vi "Scale Image.vi"(8 "error in (no error)":errorcluster, 11 "EmbedImage in":refnum<class "EmbedImage.lvclass">) -> (0 "error out":errorcluster, 3 "EmbedImage out":refnum<class "EmbedImage.lvclass">)   [LabVIEW 2023, in "EmbedImage.lvlib" / "EmbedImage.lvclass"]
uses:
  Library/EmbedImage.lvclass
  Library/EmbedImage.lvclass/EmbedImage.ctl
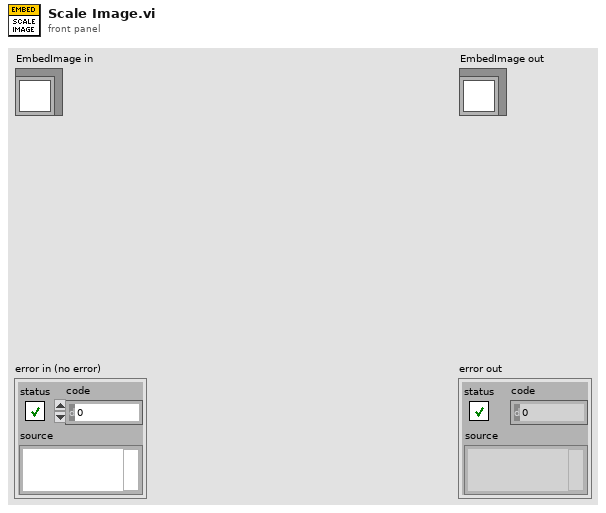
[diagram p1: front panel]
types:
  T1 = typedef "imagedata.ctl" = cluster{"image type":i32, "image depth":i32, "image":u8[], "mask":u8[], "colors":u32[], "Rectangle":cluster{"left":i16, "top":i16, "right":i16, "bottom":i16}}
  T2 = typedef "LVBoundsTypeDef.ctl" = cluster{"Width":u32, "Height":u32}
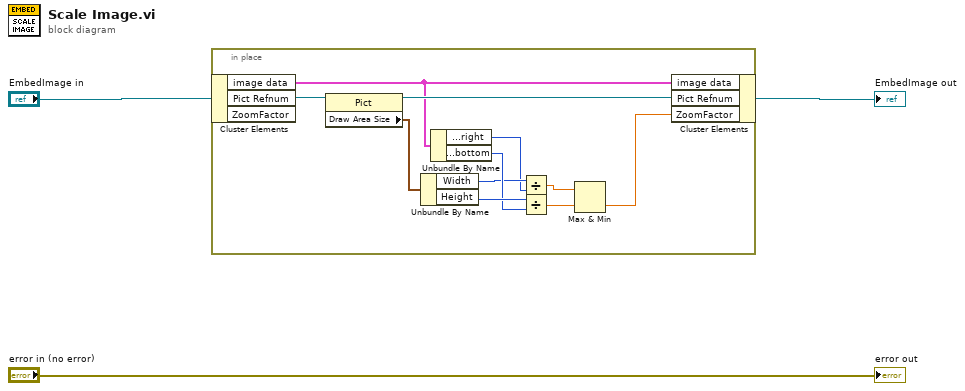
[diagram p0: block diagram]
diagram:
  n1 = in-place {
    n2 = in-place-cluster #1("EmbedImage in") -> ("image data"=w11:T1, "Pict Refnum"=w14:refnum<vi>)  [unwired: 1 out]
    n3 = property class="Pict"(reference=w14) -> (reference out=w13:refnum<vi>, "Draw Area Size"=w12:T2)  [unwired: 1 in, 1 out]
    n4 = Unbundle By Name(w12) -> ("Width"=w8:u32, "Height"=w10:u32)
    n5 = Unbundle By Name(w11) -> ("Rectangle.right"=w7:i16, "Rectangle.bottom"=w9:i16)
    n6 = Divide(x=w8, y=w7) -> (x/y=w6:dbl)
    n7 = Divide(x=w10, y=w9) -> (x/y=w5:dbl)
    n8 = Max & Min(x=w6, y=w5) -> (min(x,y)=w4:dbl)  [unwired: 1 out]
    n9 = in-place-cluster #1("image data"=w11, "Pict Refnum"=w13, "ZoomFactor"=w4) -> (→"EmbedImage out":refnum<class "EmbedImage.lvclass">)
  }
  "error out" <- "error in (no error)"
